vi "Calculate Singular Values.vi"(11 "Controllers in":T1) -> (3 "Singular Values Plot":cluster{"W":dbl[], "Magnitude":dbl[]}[](graph))   [LabVIEW 2018]
uses:
  controls/Controller.ctl
  Real-Time/Control Algorithm/Control Algorithm Selection.ctl
  <vilib>/addons/Control Design/_Model Construction/Data Typedefs.llb/CD frequency specs.ctl
  <vilib>/addons/Control Design/_Model Construction/Model Creation.llb/Model Creation SubVI/cd_Create State Space Model.vi
  <vilib>/addons/Control Design/_Model Construction/Model Information.llb/Model Information SubVIs/cd_Set Names To SS Model.vi
  <vilib>/addons/Control Design/_Model Interconnection/Model Interconnection.llb/Model Interconnection SubVI/cd_Matrix Multiply Models (SS and SS).vi
  <vilib>/addons/Control Design/_Frequency Response Analysis/Frequency Response.llb/Frequency Response subVI/cd_Singular Values (State-Space).vi
  <vilib>/addons/Control Design/_Model Construction/NI_LinSys_Model Creation.lvlib
  <vilib>/addons/Control Design/_Model Construction/NI_LinSys_Model Information.lvlib
  <vilib>/addons/Control Design/_Model Interconnection/NI_CD_Model Interconnection.lvlib
  <vilib>/addons/Control Design/_Frequency Response Analysis/NI_CD_Frequency Response.lvlib
  <vilib>/addons/Control Design/_Model Construction/NI_LinSys_Data Typedefs.lvlib
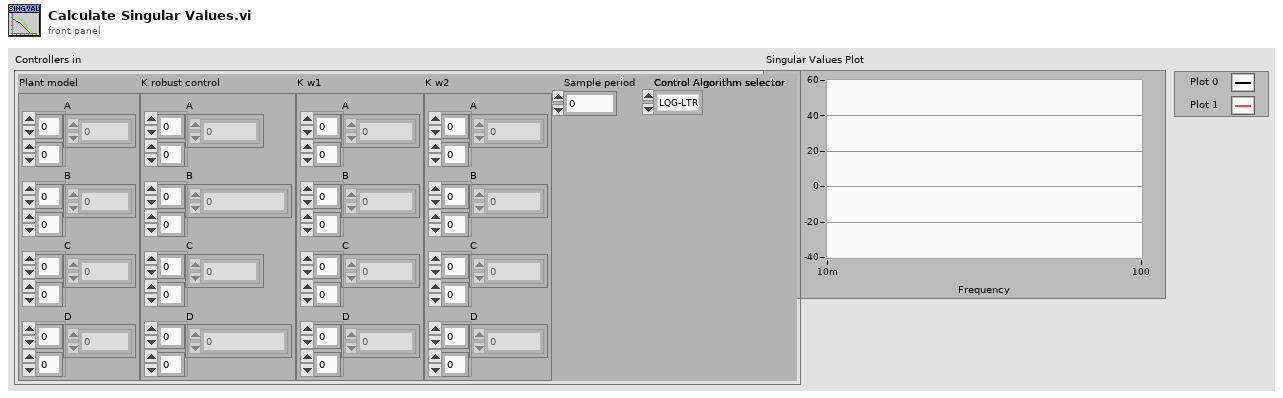
[diagram p1: front panel]
types:
  T1 = typedef "Controller.ctl" = cluster{"Plant model":cluster{"A":dbl[][], "B":dbl[][], "C":dbl[][], "D":dbl[][]}, "K robust control":cluster{"A":dbl[][], "B":dbl[][], "C":dbl[][], "D":dbl[][]}, "K w1":cluster{"A":dbl[][], "B":dbl[][], "C":dbl[][], "D":dbl[][]}, "K w2":cluster{"A":dbl[][], "B":dbl[][], "C":dbl[][], "D":dbl[][]}, "Sample period":dbl, "Control Algorithm selector":T2}
  T2 = typedef "Control Algorithm Selection.ctl" = enum16{"LQG-LTR", "Hinf"}
  T3 = typedef "NI_LinSys_Data Typedefs.lvlib/CD frequency specs.ctl" = cluster{"Initial frequency":dbl, "Final frequency":dbl, "Minimum number of points":i32, "Frequency Unit":enum16{"Hz", "rad/s"}}
  T4 = typedef "NI_LinSys_Model Typedefs.lvlib/CD State Space Model (MIMO).ctl" = cluster{"properties":T5, "A":dbl[][], "B":dbl[][], "C":dbl[][], "D":dbl[][], "StateNames":string[], "Transport Delay":dbl[][]}
  T5 = typedef "NI_LinSys_Model Typedefs.lvlib/CD General Elements.ctl" = cluster{"Model name":string, "Input names":string[], "Output names":string[], "Input Delays":dbl[], "Output Delays":dbl[], "Sampling Time":dbl, "Notes":string}
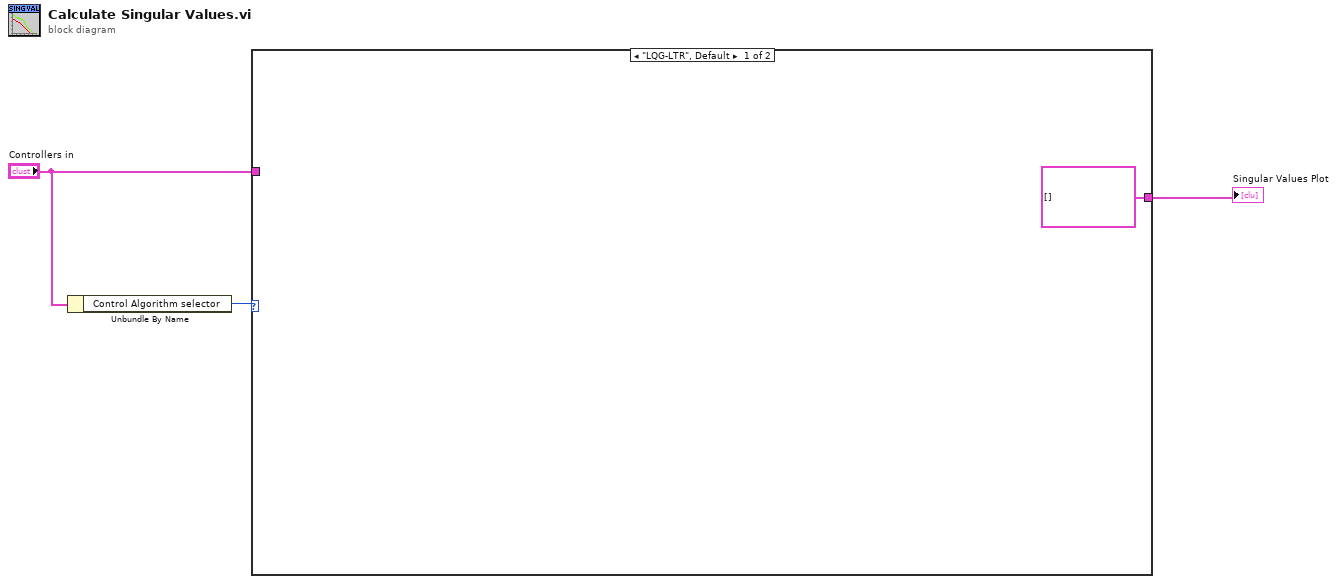
[diagram p0: block diagram]
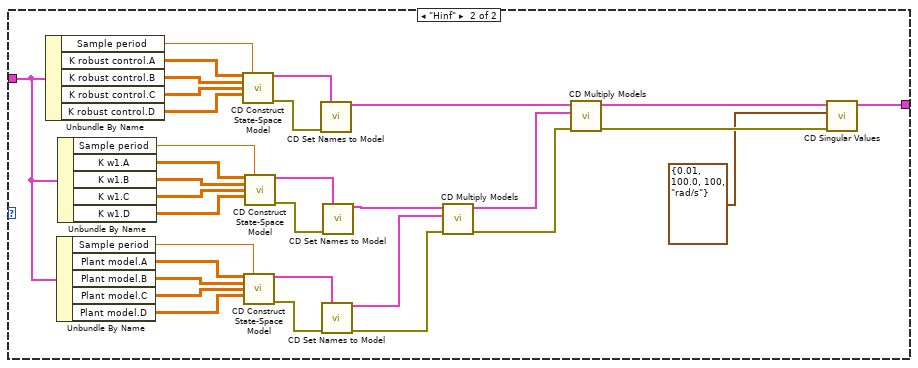
[diagram p2: hidden frame]
diagram:
  n1 = Unbundle By Name("Controllers in") -> ("Control Algorithm selector"=w1:T2)
  n2 = case shown="\"LQG-LTR\", Default" w1 {
    tunnel: [cluster{"W":dbl[], "Magnitude":dbl[]}[] [] ("Singular Values Plot") w13] -> w3
    tunnel: "Controllers in" -> [_ w5]
    frame "LQG-LTR", Default {
    }
    frame "Hinf" {
      n3 = Unbundle By Name(w5) -> ("Sample period"=w10:dbl, "K robust control.A"=w28:dbl[][], "K robust control.B"=w27:dbl[][], "K robust control.C"=w26:dbl[][], "K robust control.D"=w25:dbl[][])
      n4 = Unbundle By Name(w5) -> ("Sample period"=w12:dbl, "Plant model.A"=w21:dbl[][], "Plant model.B"=w22:dbl[][], "Plant model.C"=w23:dbl[][], "Plant model.D"=w24:dbl[][])
      n5 = Unbundle By Name(w5) -> ("Sample period"=w11:dbl, "K w1.A"=w33:dbl[][], "K w1.B"=w34:dbl[][], "K w1.C"=w35:dbl[][], "K w1.D"=w36:dbl[][])
      n6 = call-poly <vilib>:"CD Construct State-Space Model.vi"("A"=w28, "Sampling Time (s)"=w10, "B"=w27, "C"=w26, "D"=w25) -> ("State-Space Model"=w30:T4, "error out"=w29:errorcluster)  [unwired: 9 in]
      n7 = call-poly <vilib>:"CD Construct State-Space Model.vi"("A"=w21, "Sampling Time (s)"=w12, "B"=w22, "C"=w23, "D"=w24) -> ("State-Space Model"=w19:T4, "error out"=w20:errorcluster)  [unwired: 9 in]
      n8 = call-poly <vilib>:"CD Construct State-Space Model.vi"("A"=w33, "Sampling Time (s)"=w11, "B"=w34, "C"=w35, "D"=w36) -> ("State-Space Model"=w31:T4, "error out"=w32:errorcluster)  [unwired: 9 in]
      n9 = call-poly <vilib>:"CD Set Names to Model.vi"("State-Space Model In"=w30, "error in (no error)"=w29) -> ("Model Out"=w15:T4)  [unwired: 12 in, 1 out]
      n10 = call-poly <vilib>:"CD Set Names to Model.vi"("State-Space Model In"=w19, "error in (no error)"=w20) -> ("Model Out"=w17:T4, "error out"=w7:errorcluster)  [unwired: 12 in]
      n11 = call-poly <vilib>:"CD Set Names to Model.vi"("State-Space Model In"=w31, "error in (no error)"=w32) -> ("Model Out"=w18:T4)  [unwired: 12 in, 1 out]
      n12 = call-poly <vilib>:"CD Multiply Models.vi"("error in (no error)"=w7, "Model 2"=w17, "Model 1"=w18) -> ("error out"=w8:errorcluster, "Model Out"=w16:T4)  [unwired: 7 in]
      n13 = call-poly <vilib>:"CD Multiply Models.vi"("error in (no error)"=w8, "Model 2"=w16, "Model 1"=w15) -> ("error out"=w9:errorcluster, "Model Out"=w14:T4)  [unwired: 7 in]
      n14 = call-poly <vilib>:"CD Singular Values.vi"("error in (no error)"=w9, "Frequency Range"=T3 {"Initial frequency"=0.01, "Final frequency"=100.0, "Minimum number of points"=100, "Frequency Unit"=enum."rad/s"}, "State-Space Model"=w14) -> ("Singular Values Plot"=w13:cluster{"W":dbl[], "Magnitude":dbl[]}[])  [unwired: 6 in, 2 out]
    }
  }
  "Singular Values Plot" <- w3
